vi "LimeLight_PID.vi"(9 "Numeric 2":dbl, 10 "Numeric":dbl) -> (1 "output_ty":dbl, 2 "output_tx":dbl)   [LabVIEW 2020]
uses:
  GlobalVariables.vi
  <vilib>/functionblocks/Control/PID/PID.vi
  <vilib>/functionblocks/FB Core/FB Core.xnode
  <vilib>/functionblocks/NI_FunctionBlock Libraries.lvlib
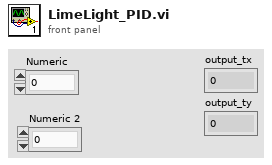
[diagram p1: front panel]
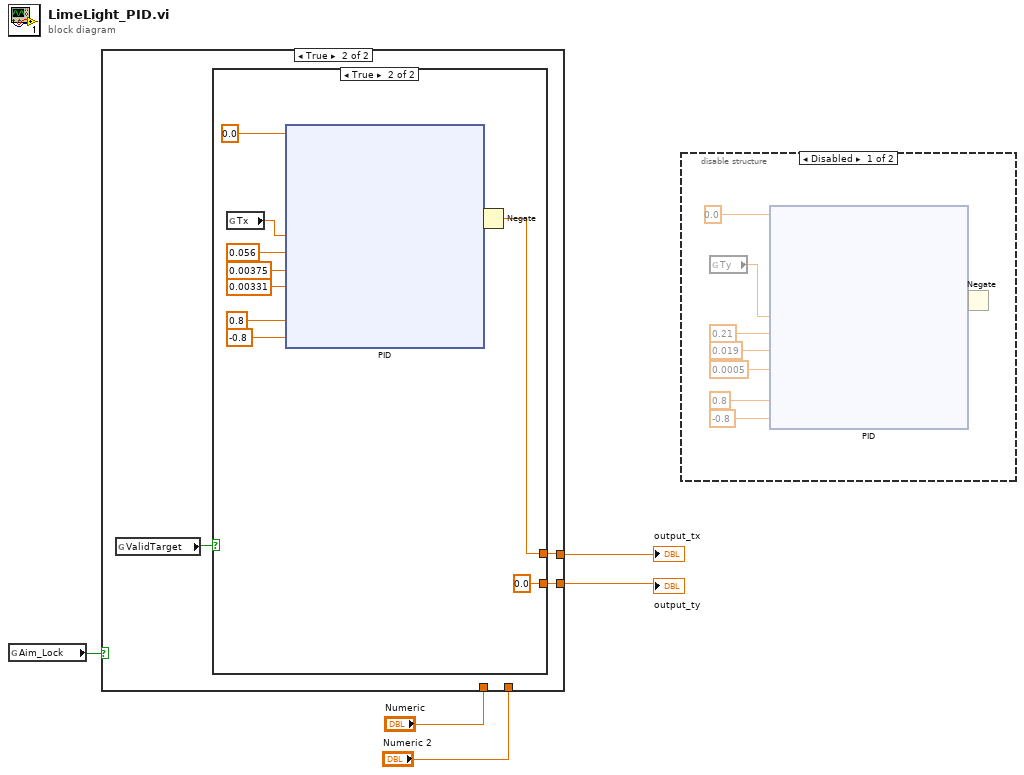
[diagram p0: block diagram]
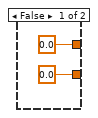
[diagram p4: hidden frame]
diagram:
  n1 = global read "GlobalVariables.vi" "Aim_Lock"() -> (w5:bool)
  n2 = case shown="True" w5 {
    tunnel: [w6 w9] -> w3
    tunnel: [w7 w10] -> w4
    tunnel: "Numeric" -> [w7 _]
    tunnel: "Numeric 2" -> [w6 _]
    frame False {
    }
    frame True {
      n3 = global read "GlobalVariables.vi" "ValidTarget"() -> (w8:bool)
      n4 = case shown="True" w8 {
        tunnel: [0.0 ("x+y") w22] -> w10
        tunnel: [0.0 ("x+y") 0.0 ("x+y")] -> w9
        frame False {
        }
        frame True {
          n5 = global read "GlobalVariables.vi" "Tx"() -> (w20:dbl)
          n6 = xnode "PID"("setpoint"=0.0, "process variable"=w20, "proportional gain (Kc)"=0.056, "integral time (Ti, min)"=0.00375, "derivative time (Td, min)"=0.00331, "output high"=0.8, "output low"=-0.8) -> ("output"=w19:dbl)  [unwired: 2 in, 1 out]
          n7 = Negate(x=w19) -> (-x=w22:dbl)
        }
      }
    }
  }
  "output_tx" <- w4
  "output_ty" <- w3
  n8 = disable-structure shown="Disabled" {
    frame Disabled {
      n9 = global read "GlobalVariables.vi" "Ty"() -> (w92:dbl)
      n10 = xnode "PID"("setpoint"=0.0, "process variable"=w92, "proportional gain (Kc)"=0.21, "integral time (Ti, min)"=0.019, "derivative time (Td, min)"=0.0005, "output high"=0.8, "output low"=-0.8) -> ("output"=w94:dbl)  [unwired: 2 in, 1 out]
      n11 = Negate(x=w94) -> (-x=w95:dbl)
    }
    frame Enabled {
    }
  }
